vi "Detect Shape (Main).vi"() -> ()   [LabVIEW 2014]
doc: "Very simple example showing how to use the base VIs to control the AR Drone and receive and display video data."
uses:
  Global.vi
  <vilib>/vision/NI_Vision_Development_Module.lvlib
panel:
  in  "File Path":path=path "E:/Dropbox/UTCN/Summer 2015/DroneMainRepo/TESTING/Vision & Image Processing/Templates (images)/new sample.png"
  in  "Rotation Angle Ranges (degrees)":cluster{sgl, sgl}[](array[cluster])=[{-90.0, 90.0}] {"?" format="%.2f"; "?" format="%.2f"}
  out "Matches[0]":T1
  out "Get video error":errorcluster
  out "Output image":T2(plugin-control)
  in  "milliseconds to wait":u32
  out "delay":u32=31
  in  "stop":bool
  out "Video processing error":errorcluster={"status"=TRUE, "code"=-1074395395, "source"="IMAQ Learn Color Pattern\n  "}
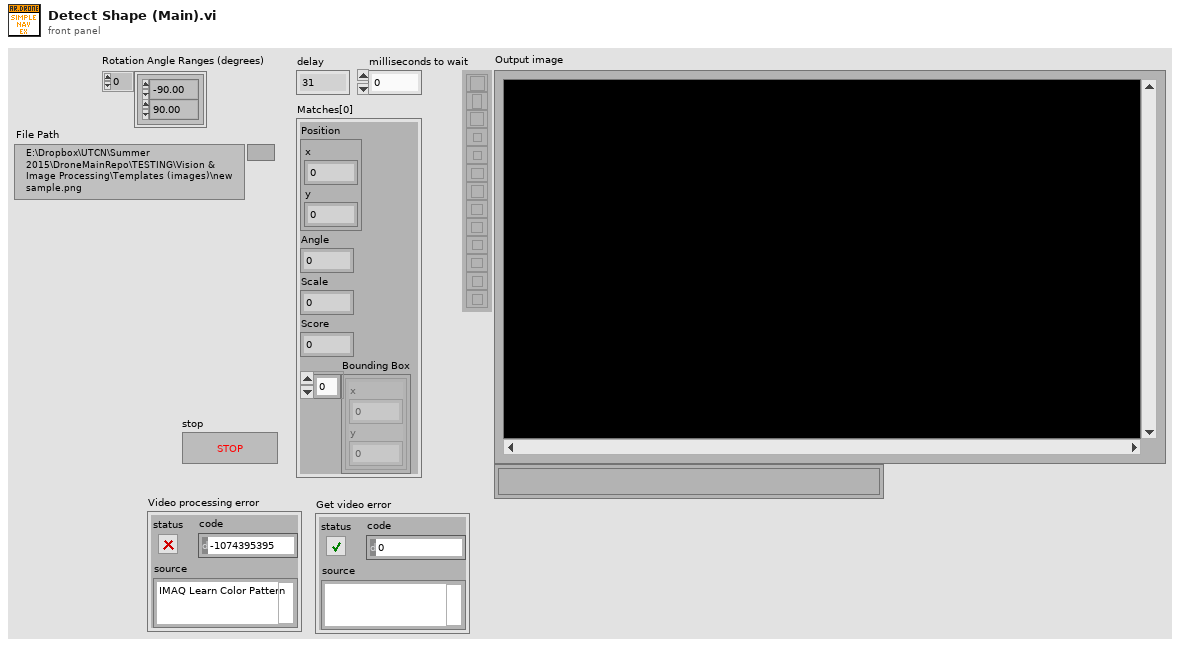
[diagram p1: front panel]
types:
  T1 = cluster{"Position":cluster{"x":sgl, "y":sgl}, "Angle":sgl, "Scale":sgl, "Score":sgl, "Bounding Box":cluster{"x":sgl, "y":sgl}[]}
  T2 = typedef "IMAQ Image.ctl" = refnum<image>
  T3 = cluster{"Position":cluster{"x":sgl, "y":sgl}, "Angle":sgl, "Scale":sgl, "Score":sgl, "Bounding Box":cluster{"x":sgl, "y":sgl}[]}[]
  T4 = cluster{"Matches[0]":cluster{"Position":cluster{"x":sgl, "y":sgl}, "Angle":sgl, "Scale":sgl, "Score":sgl, "Bounding Box":cluster{"x":sgl, "y":sgl}[]}, "Matches[1]":cluster{"Position":cluster{"x":sgl, "y":sgl}, "Angle":sgl, "Scale":sgl, "Score":sgl, "Bounding Box":cluster{"x":sgl, "y":sgl}[]}, "Matches[2]":cluster{"Position":cluster{"x":sgl, "y":sgl}, "Angle":sgl, "Scale":sgl, "Score":sgl, "Bounding Box":cluster{"x":sgl, "y":sgl}[]}, "Matches[3]":cluster{"Position":cluster{"x":sgl, "y":sgl}, "Angle":sgl, "Scale":sgl, "Score":sgl, "Bounding Box":cluster{"x":sgl, "y":sgl}[]}, "Matches[4]":cluster{"Position":cluster{"x":sgl, "y":sgl}, "Angle":sgl, "Scale":sgl, "Score":sgl, "Bounding Box":cluster{"x":sgl, "y":sgl}[]}, "Matches[5]":cluster{"Position":cluster{"x":sgl, "y":sgl}, "Angle":sgl, "Scale":sgl, "Score":sgl, "Bounding Box":cluster{"x":sgl, "y":sgl}[]}, "Matches[6]":cluster{"Position":cluster{"x":sgl, "y":sgl}, "Angle":sgl, "Scale":sgl, "Score":sgl, "Bounding Box":cluster{"x":sgl, "y":sgl}[]}, "Matches[7]":cluster{"Position":cluster{"x":sgl, "y":sgl}, "Angle":sgl, "Scale":sgl, "Score":sgl, "Bounding Box":cluster{"x":sgl, "y":sgl}[]}, "Matches[8]":cluster{"Position":cluster{"x":sgl, "y":sgl}, "Angle":sgl, "Scale":sgl, "Score":sgl, "Bounding Box":cluster{"x":sgl, "y":sgl}[]}}
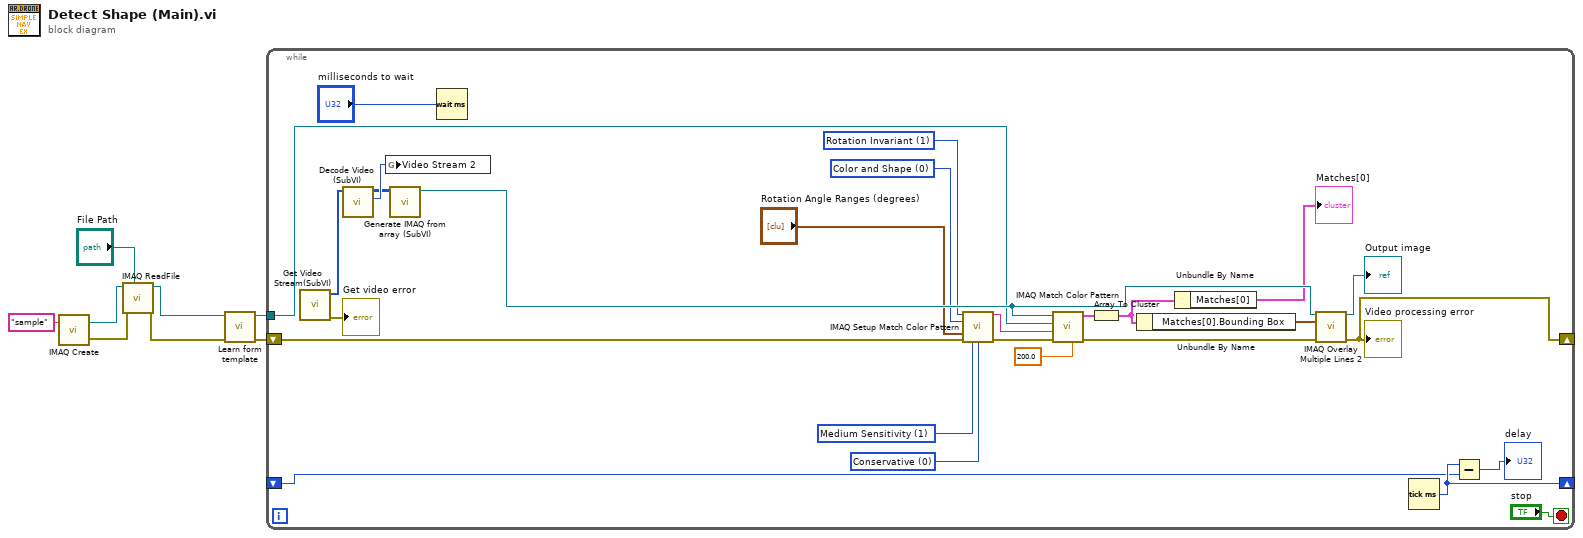
[diagram p0: block diagram]
diagram:
  n1 = call "IMAQ Create"("Image Name"="sample") -> ("New Image"=w5:T2, "error out"=w2:errorcluster)  [unwired: 4 in]
  n2 = call "IMAQ ReadFile"("File Path"="File Path", "error in (no error)"=w2, "Image"=w5) -> ("error out"=w1:errorcluster, "Image Out"=w3:T2)  [unwired: 4 in, 3 out]
  n3 = call "Learn form template.vi"("error in (no error)"=w1, "Template Image"=w3) -> ("error out"=w8:errorcluster, "Refnum out"=w7:T2)  [unwired: 8 in]
  n4 = while {
    shift-right: [w31] -> _
    shift-left: _ -> [w30]
    shift-right: [w24] -> _
    shift-left: w8 -> [w27]
    tunnel: w7 -> [w22]
    stop <- "stop" stop-if-true
    w10 = u32 1 items=["Low Sensitivity", "Medium Sensitivity", "High Sensitivity"] ("Color Sensitivity")
    w11 = u32 0 items=["Conservative", "Balance", "Aggressive", "Very Aggressive"] ("Search Strategy")
    w12 = u32 0 items=["Color and Shape", "Color", "Shape"] ("Match Feature Mode")
    w13 = u32 1 items=["Shift Invariant", "Rotation Invariant"] ("Match Mode")
    n5 = call "Get Video Stream(SubVI).vi"() -> ("error out"=→"Get video error":errorcluster, "ImgData"=w35:u8[])  [unwired: 10 in]
    n6 = call "Decode Video (SubVI).vi"("ImgData"=w35) -> ("new picture"=w34:picture, "Array"=w33:u32[][])  [unwired: 9 in]
    n7 = global write "Global.vi" "Video Stream 2"(w34) -> ()
    n8 = call "Generate IMAQ from array (SubVI).vi"("Array"=w33) -> ("Refnum out"=w25:T2)  [unwired: 10 in]
    n9 = Wait (ms)(milliseconds to wait="milliseconds to wait") -> ()  [unwired: 1 out]
    n10 = call "IMAQ Setup Match Color Pattern"("Match Mode"=w13, "Match Feature Mode"=w12, "Rotation Angle Ranges (degrees)"="Rotation Angle Ranges (degrees)", "error in (no error)"=w27, "Color Sensitivity"=w10, "Search Strategy"=w11) -> ("Match Color Pattern Setup Data"=w20:string, "error out"=w21:errorcluster)  [unwired: 8 in]
    n11 = call "IMAQ Match Color Pattern"("Minimum Match Score"=sgl 200.0, "error in (no error)"=w21, "Match Color Pattern Setup Data"=w20, "Template Image"=w22, "Image"=w25) -> ("error out"=w17:errorcluster, "Matches"=w19:T3)  [unwired: 4 in, 1 out]
    n12 = Array To Cluster(array=w19) -> (cluster=w15:T4)
    n13 = Unbundle By Name(w15) -> ("Matches[0].Bounding Box"=w18:cluster{"x":sgl, "y":sgl}[])
    n14 = Unbundle By Name(w15) -> ("Matches[0]"=→"Matches[0]":T1)
    n15 = call "IMAQ Overlay Multiple Lines 2"("Image"=w25, "Line End Points"=w18, "error in (no error)"=w17) -> ("Image Out"=→"Output image":T2, "error out"=w24:errorcluster)  [unwired: 11 in]
    "Video processing error" <- w24
    n16 = Tick Count (ms)() -> (millisecond timer value=w31:u32)
    n17 = Subtract(x=w31, y=w30) -> (x-y=→"delay":u32)
  }
